vi "StopMoteurs.vi"   [LabVIEW 2017]
uses:
  ICNC/ICNC2.lvlib
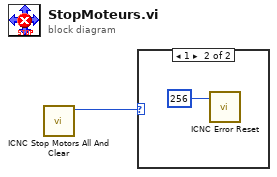
[diagram p0: block diagram]
diagram:
  n1 = call "ICNC Stop Motors All And Clear.vi"() -> ("function return"=w1:u32)  [unwired: 10 in, 1 out]
  n2 = case shown="1" w1 {
    frame 0, Default {
    }
    frame 1 {
      n3 = call "ICNC Error Reset.vi"("ErrorBits"=256) -> ()  [unwired: 9 in, 2 out]
    }
  }
